vi "myDAQ source.vi"() -> ()   [LabVIEW 2015]
uses:
  <vilib>/DAQmx/write.llb/DAQmx Write (Analog 1D Wfm NChan NSamp).vi
  <vilib>/DAQmx/create/channels.llb/DAQmx Create Channel (AO-Voltage-Basic).vi
  <vilib>/DAQmx/configure/timing.llb/DAQmx Timing (Sample Clock).vi
  <vilib>/DAQmx/miscellaneous.llb/DAQmx Fill In Error Info.vi
  <vilib>/measure/NI_MABase.lvlib
  <resource>/objmgr/daqmx.rc
panel:
  out "Waveform Graph":waveform(dbl)[](graph)
  in  "AO1":T1={"Waveform Type"=enum."Sine Wave", "Frequency (Hz)"=50.0, "Amplitude (V)"=1.0, "Offset (V)"=2.5, "Phase (Deg)"=90.0} {"Phase (Deg)" format="%.2p"; "Offset (V)" format="%0.2p"; "Amplitude (V)" format="%0.2p"; "Frequency (Hz)" format="%0.2p"}
  in  "AO0":T1={"Waveform Type"=enum."Sine Wave", "Frequency (Hz)"=20.0, "Amplitude (V)"=1.0, "Offset (V)"=2.5, "Phase (Deg)"=0.0} {"Phase (Deg)" format="%.2p"; "Offset (V)" format="%0.2p"; "Amplitude (V)" format="%0.2p"; "Frequency (Hz)" format="%0.2p"}
  in  "Stop":bool
  in  "Number of Samples":i32=1000
  in  "Sample Clock Source":tag="OnboardClock"
  in  "Sample Rate":dbl=1000.0
  in  "Physical Channel(s)":tag="myDAQ1/ao0:1"
  in  "Min Voltage":dbl=-5.0
  in  "Max Voltage":dbl=5.0
  # "myDAQ AO Function Generator"
  # "Created by zxlee (iamzxlee.wordpress.com)"
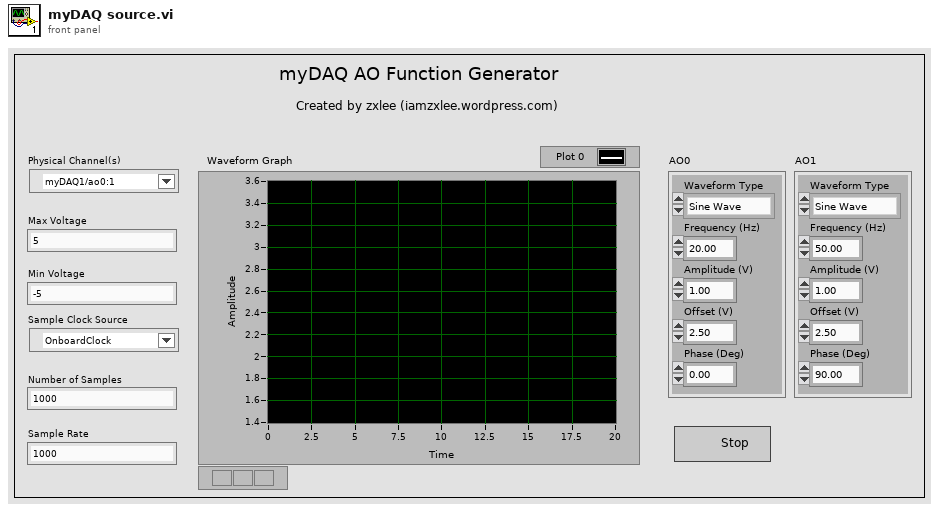
[diagram p1: front panel]
types:
  T1 = cluster{"Waveform Type":enum16{"Sine Wave", "Triangle Wave", "Square Wave", "Sawtooth Wave"}, "Frequency (Hz)":dbl, "Amplitude (V)":dbl, "Offset (V)":dbl, "Phase (Deg)":dbl}
  T2 = cluster{"Waveform Type":enum16{"Sine Wave", "Triangle Wave", "Square Wave", "Sawtooth Wave"}, "Frequency (Hz)":dbl, "Amplitude (V)":dbl, "Offset (V)":dbl, "Phase (Deg)":dbl}[]
  T3 = enum16{"Sine Wave", "Triangle Wave", "Square Wave", "Sawtooth Wave"}
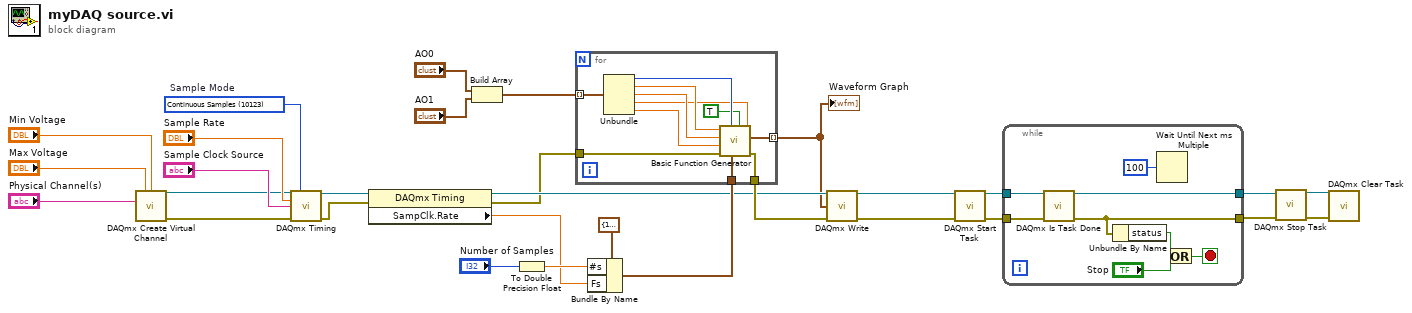
[diagram p0: block diagram]
diagram:
  w7 = 10123 items=["Finite Samples"=10178, "Continuous Samples"=10123, "Hardware Timed Single Point"=12522]  # Sample Mode
  n1 = call-poly <vilib>:"DAQmx Create Virtual Channel.vi"("maximum value"="Max Voltage", "minimum value"="Min Voltage", "physical channels"="Physical Channel(s)") -> ("task out"=w14:refnum<k21>, "error out"=w13:errorcluster)  [unwired: 11 in]
  n2 = call-poly <vilib>:"DAQmx Timing.vi"("task/channels in"=w14, "sample mode"=w7, "rate"="Sample Rate", "source"="Sample Clock Source", "error in"=w13) -> ("task out"=w6:refnum<k21>, "error out"=w4:errorcluster)  [unwired: 9 in]
  n3 = property class="DAQmx Timing"(reference=w6, error in=w4) -> (reference out=w5:refnum<k21>, error out=w3:errorcluster, "SampClk.Rate"=w2:dbl)
  n4 = Build Array("AO0", "AO1") -> (w10:T2)
  n5 = To Double Precision Float(number="Number of Samples") -> (double precision float=w24:dbl)
  n6 = Bundle By Name(cluster=cluster{"Fs":dbl, "#s":dbl} {"Fs"=1000.0, "#s"=1000.0} ("sampling info"), "#s"=w24, "Fs"=w2) -> (w22:cluster{"Fs":dbl, "#s":dbl})
  n7 = for {
    tunnel: w3 -> [w41]
    tunnel: w22 -> [w40]
    tunnel: [w39] -> w23
    tunnel: [w38] -> w1 mode=indexing
    tunnel: w10 -> [w37] mode=indexing
    n8 = Unbundle(w37) -> ("Waveform Type"=w36:T3, "Frequency (Hz)"=w35:dbl, "Amplitude (V)"=w34:dbl, "Offset (V)"=w33:dbl, "Phase (Deg)"=w32:dbl)
    n9 = call <vilib>:"Basic Function Generator.vi"("offset"=w33, "reset signal"=TRUE, "sampling info"=w40, "signal type"=w36, "error in (no error)"=w41, "phase"=w32, "amplitude"=w34, "frequency"=w35) -> ("error out"=w39:errorcluster, "signal out"=w38:waveform(dbl))  [unwired: 1 in, 1 out]
  }
  "Waveform Graph" <- w1
  n10 = call-poly <vilib>:"DAQmx Write.vi"("task/channels in"=w5, "data"=w1, "error in"=w23) -> ("task out"=w9:refnum<k21>, "error out"=w8:errorcluster)  [unwired: 10 in, 1 out]
  n11 = call <vilib>:"DAQmx Start Task.vi"("task/channels in"=w9, "error in"=w8) -> ("task out"=w20:refnum<k21>, "error out"=w19:errorcluster)  [unwired: 12 in]
  n12 = while {
    tunnel: w20 -> [w49]
    tunnel: w19 -> [w48]
    tunnel: [w45] -> w15
    tunnel: [w46] -> w16
    stop <- w47 stop-if-true
    n13 = call <vilib>:"DAQmx Is Task Done.vi"("task/channels in"=w49, "error in"=w48) -> ("task out"=w46:refnum<k21>, "error out"=w45:errorcluster)  [unwired: 11 in, 1 out]
    n14 = Unbundle By Name(w45) -> ("status"=w44:bool)
    n15 = Wait Until Next ms Multiple(millisecond multiple=u32 100) -> ()  [unwired: 1 out]
    n16 = Or(x=w44, y="Stop") -> (x .or. y?=w47:bool)
  }
  n17 = call <vilib>:"DAQmx Stop Task.vi"("task/channels in"=w16, "error in"=w15) -> ("task out"=w18:refnum<k21>, "error out"=w17:errorcluster)  [unwired: 12 in]
  n18 = call <vilib>:"DAQmx Clear Task.vi"("task in"=w18, "error in"=w17) -> ()  [unwired: 13 in, 1 out]
